vi "Digital_Bridge_3_kart.vi"() -> ()   [LabVIEW 2014] (continued)
                      frame True {
                        n3554 = local read "Frekanslar"() -> (w1876:dbl[])
                        n3555 = Array Size(array=w1876) -> (size(s)=w1875:i32)
                        n3556 = local read "frekans index"() -> (w1877:dbl)
                        n3557 = Decrement(x=w1875) -> (x-1=w1874:i32)
                        n3558 = Equal?(x=w1877, y=w1874) -> (x = y?=w1878:bool)
                        n3559 = case shown="False" w1878 {
                          tunnel: w1877 -> [w1879 w1891]
                          frame False {
                            n3560 = flat-sequence {
                              tunnel: w1879 -> [w1881]
                              frame #0 {
                                n3561 = local read "control hz array"() -> (w1883:dbl[][])
                                n3562 = call "change2d.vi"("reset(default false)"=FALSE, "index (col)"=w1881, "index (row)"=3, "read/write(T/F)"=FALSE, "2D Array"=w1883) -> ("2D Array Result"=w1882:dbl[][])  [unwired: 5 in, 1 out]
                                n3563 = local write "control hz array"(w1882) -> ()
                              }
                              frame #1 {
                                n3564 = local read "frekans index"() -> (w1890:dbl)
                                n3565 = local write "default input"(TRUE ("default values 2")) -> ()
                                n3566 = Increment(x=w1890) -> (x+1=w1889:dbl)
                                n3567 = local write "continue"(FALSE ("continue")) -> ()
                                n3568 = local write "error 2"(FALSE ("continue")) -> ()
                                n3569 = local write "frekans index"(w1889) -> ()
                              }
                            }
                          }
                          frame True {
                            n3570 = flat-sequence {
                              tunnel: w1891 -> [w1893]
                              frame #0 {
                                n3571 = local read "control hz array"() -> (w1895:dbl[][])
                                n3572 = call "change2d.vi"("reset(default false)"=FALSE, "index (col)"=w1893, "index (row)"=3, "read/write(T/F)"=FALSE, "2D Array"=w1895) -> ("2D Array Result"=w1894:dbl[][])  [unwired: 5 in, 1 out]
                                n3573 = local write "control hz array"(w1894) -> ()
                              }
                              frame #1 {
                                n3574 = local write "frekans index"(0.0 ("frekans index")) -> ()
                                n3575 = local write "default input"(TRUE ("default values 2")) -> ()
                                n3576 = local write "continue"(FALSE ("continue")) -> ()
                                n3577 = local write "error 2"(FALSE ("continue")) -> ()
                              }
                            }
                          }
                        }
                      }
                    }
                  }
                  frame True {
                    n3578 = local read "Frekanslar"() -> (w1904:dbl[])
                    n3579 = local read "frekans index"() -> (w1906:dbl)
                    n3580 = Array Size(array=w1904) -> (size(s)=w1903:i32)
                    n3581 = Decrement(x=w1903) -> (x-1=w1902:i32)
                    n3582 = Equal?(x=w1906, y=w1902) -> (x = y?=w1905:bool)
                    n3583 = case shown="True" w1905 {
                      frame False {
                        n3584 = flat-sequence {
                          frame #0 {
                            n3585 = local read "frekans index"() -> (w1908:dbl)
                            n3586 = Increment(x=w1908) -> (x+1=w1907:dbl)
                            n3587 = local write "frekans index"(w1907) -> ()
                          }
                          frame #1 {
                            n3588 = local write "default input"(TRUE ("default values 2")) -> ()
                            n3589 = local write "continue"(FALSE ("continue")) -> ()
                          }
                          frame #2 {
                            n3590 = local write "pass hz"(FALSE ("pass hz")) -> ()
                          }
                          frame #3 {
                          }
                        }
                      }
                      frame True {
                        n3591 = flat-sequence {
                          frame #0 {
                            n3592 = local write "frekans index"(0.0 ("frekans index")) -> ()
                          }
                          frame #1 {
                            n3593 = local write "default input"(TRUE ("default values 2")) -> ()
                            n3594 = local write "continue"(FALSE ("continue")) -> ()
                          }
                          frame #2 {
                            n3595 = local write "pass hz"(FALSE ("pass hz")) -> ()
                          }
                          frame #3 {
                          }
                        }
                      }
                    }
                  }
                }
              }
              frame #2 {
                w1916 = 0.0 ("amplitude 2/0")
                w1918 = 0.0 ("result output x [Wagner]")
                w1920 = FALSE ("Boolean 5")
                w1921 = FALSE
                w1922 = FALSE
                n3596 = case shown="True" "default input" {
                  frame False {
                  }
                  frame True {
                    n3597 = flat-sequence {
                      frame #0 {
                        w1936 = 0.0 ("iterasyon ana denge")
                        w1935 = 0.0 ("iterasyon ana denge")
                        w1934 = 0.0 ("iterasyon ana denge")
                        w1933 = 0.0 ("iterasyon ana denge")
                        w1932 = 0.0 ("iterasyon ana denge")
                        # "Frekans a göre iterasyon x algıla ona gore faz alınacak"
                        n3598 = global read "First_input_values.vi" "Active"() -> (w1923:bool)
                        n3599 = local read "frekans index"() -> (w1930:dbl)
                        n3600 = local read "control hz array"() -> (w1927:dbl[][])
                        n3601 = local write "output 1 y [10R]"(w1936) -> ()
                        n3602 = local write "input 1 y [10R]"(w1936) -> ()
                        n3603 = local write "output 2 y [10R]"(w1936) -> ()
                        n3604 = local write "input 2 y [10R]"(w1936) -> ()
                        n3605 = local write "input 2 x [10R]"(w1936) -> ()
                        n3606 = local write "output 2 x [10R]"(w1936) -> ()
                        n3607 = local write "input 1 x [10R]"(w1936) -> ()
                        n3608 = local write "output 1 x [10R]"(w1936) -> ()
                        n3609 = call "change2d.vi"("reset(default false)"=FALSE, "index (col)"=w1930, "index (row)"=3, "read/write(T/F)"=TRUE, "2D Array"=w1927) -> ("result count"=w1926:dbl)  [unwired: 5 in, 1 out]
                        n3610 = case shown="True" w1923 {
                          frame False {
                            n3611 = global read "First_input_values.vi" "X 1. input W"() -> (w1979:dbl)
                            n3612 = global read "First_input_values.vi" "X 2. input W"() -> (w1980:dbl)
                            n3613 = global read "First_input_values.vi" "X 1. input W"() -> (w1984:dbl)
                            n3614 = global read "First_input_values.vi" "X 2. input W"() -> (w1983:dbl)
                            n3615 = global read "First_input_values.vi" "Y 1. input W"() -> (w1981:dbl)
                            n3616 = global read "First_input_values.vi" "Y 2. input W"() -> (w1982:dbl)
                            n3617 = global read "First_input_values.vi" "Y 1. input W"() -> (w1986:dbl)
                            n3618 = global read "First_input_values.vi" "Y 2. input W"() -> (w1985:dbl)
                            n3619 = global read "First_input_values.vi" "X 1. input KV"() -> (w1971:dbl)
                            n3620 = global read "First_input_values.vi" "X 2. input KV"() -> (w1972:dbl)
                            n3621 = global read "First_input_values.vi" "X 1. input KV"() -> (w1976:dbl)
                            n3622 = global read "First_input_values.vi" "X 2. input KV"() -> (w1975:dbl)
                            n3623 = global read "First_input_values.vi" "Y 1. input KV"() -> (w1973:dbl)
                            n3624 = global read "First_input_values.vi" "Y 2. input KV"() -> (w1974:dbl)
                            n3625 = global read "First_input_values.vi" "Y 1. input KV"() -> (w1978:dbl)
                            n3626 = global read "First_input_values.vi" "Y 2. input KV"() -> (w1977:dbl)
                            n3627 = local write "Wagner Xk"(w1979) -> ()
                            n3628 = local write "Wagner  X(k-1)"(w1980) -> ()
                            n3629 = local write "X 1.input W"(w1984) -> ()
                            n3630 = local write "X 2.input W"(w1983) -> ()
                            n3631 = local write "Wagner Yk"(w1981) -> ()
                            n3632 = local write "Wagner Y(k-1)"(w1982) -> ()
                            n3633 = local write "Y 1.input W"(w1986) -> ()
                            n3634 = local write "Y 2.input W"(w1985) -> ()
                            n3635 = local write "Kelvin Xk"(w1971) -> ()
                            n3636 = local write "Kelvin X(k-1)"(w1972) -> ()
                            n3637 = local write "X 1.input KV"(w1976) -> ()
                            n3638 = local write "X 2.input KV"(w1975) -> ()
                            n3639 = local write "Kelvin Yk"(w1973) -> ()
                            n3640 = local write "Kelvin Y(k-1)"(w1974) -> ()
                            n3641 = local write "Y 1.input KV"(w1978) -> ()
                            n3642 = local write "Y 2.input KV"(w1977) -> ()
                            n3643 = global read "First_input_values.vi" "X 1. input AD"() -> (w1963:dbl)
                            n3644 = global read "First_input_values.vi" "X 2. input AD"() -> (w1964:dbl)
                            n3645 = global read "First_input_values.vi" "X 1. input AD"() -> (w1968:dbl)
                            n3646 = global read "First_input_values.vi" "X 2. input AD"() -> (w1967:dbl)
                            n3647 = global read "First_input_values.vi" "Y 1. input AD"() -> (w1965:dbl)
                            n3648 = global read "First_input_values.vi" "Y 2. input AD"() -> (w1966:dbl)
                            n3649 = global read "First_input_values.vi" "Y 1. input AD"() -> (w1970:dbl)
                            n3650 = global read "First_input_values.vi" "Y 2. input AD"() -> (w1969:dbl)
                            n3651 = global read "First_input_values.vi" "X 1. input 10R"() -> (w1955:dbl)
                            n3652 = global read "First_input_values.vi" "X 2. input 10R"() -> (w1956:dbl)
                            n3653 = global read "First_input_values.vi" "Y 1. input 10R"() -> (w1957:dbl)
                            n3654 = global read "First_input_values.vi" "Y 2. input 10R"() -> (w1958:dbl)
                            n3655 = global read "First_input_values.vi" "X 1. input 10R"() -> (w1960:dbl)
                            n3656 = global read "First_input_values.vi" "X 2. input 10R"() -> (w1959:dbl)
                            n3657 = global read "First_input_values.vi" "Y 1. input 10R"() -> (w1962:dbl)
                            n3658 = global read "First_input_values.vi" "Y 2. input 10R"() -> (w1961:dbl)
                            n3659 = local write "AD Xk"(w1963) -> ()
                            n3660 = local write "AD X(k-1)"(w1964) -> ()
                            n3661 = local write "X 1.input AD"(w1968) -> ()
                            n3662 = local write "X 2.input AD"(w1967) -> ()
                            n3663 = local write "AD Yk"(w1965) -> ()
                            n3664 = local write "AD Y(k-1)"(w1966) -> ()
                            n3665 = local write "Y 1.input AD"(w1970) -> ()
                            n3666 = local write "Y 2.input AD"(w1969) -> ()
                            n3667 = local write "10R Xk"(w1955) -> ()
                            n3668 = local write "10R X(k-1)"(w1956) -> ()
                            n3669 = local write "X 1.input 10R"(w1960) -> ()
                            n3670 = local write "X 2.input 10R"(w1959) -> ()
                            n3671 = local write "10R Yk"(w1957) -> ()
                            n3672 = local write "10R Y(k-1)"(w1958) -> ()
                            n3673 = local write "Y 1.input 10R"(w1962) -> ()
                            n3674 = local write "Y 2.input 10R"(w1961) -> ()
                            n3675 = global read "First_input_values.vi" "X 1. input 1R"() -> (w1947:dbl)
                            n3676 = global read "First_input_values.vi" "X 2. input 1R"() -> (w1948:dbl)
                            n3677 = global read "First_input_values.vi" "X 1. input 1R"() -> (w1952:dbl)
                            n3678 = global read "First_input_values.vi" "X 2. input 1R"() -> (w1951:dbl)
                            n3679 = global read "First_input_values.vi" "Y 1. input 1R"() -> (w1949:dbl)
                            n3680 = global read "First_input_values.vi" "Y 2. input 1R"() -> (w1950:dbl)
                            n3681 = global read "First_input_values.vi" "Y 1. input 1R"() -> (w1954:dbl)
                            n3682 = global read "First_input_values.vi" "Y 2. input 1R"() -> (w1953:dbl)
                            n3683 = global read "First_input_values.vi" "Y range 10R"() -> (w1945:dbl)
                            n3684 = global read "First_input_values.vi" "Y range AD"() -> (w1946:dbl)
                            n3685 = global read "First_input_values.vi" "X range 10R"() -> (w1940:dbl)
                            n3686 = global read "First_input_values.vi" "Y range KV"() -> (w1942:dbl)
                            n3687 = global read "First_input_values.vi" "Y range 1R"() -> (w1944:dbl)
                            n3688 = global read "First_input_values.vi" "X range AD"() -> (w1941:dbl)
                            n3689 = global read "First_input_values.vi" "Y range W"() -> (w1943:dbl)
                            n3690 = global read "First_input_values.vi" "X range KV"() -> (w1937:dbl)
                            n3691 = global read "First_input_values.vi" "X range 1R"() -> (w1939:dbl)
                            n3692 = global read "First_input_values.vi" "X range W"() -> (w1938:dbl)
                            n3693 = local write "1R Xk"(w1947) -> ()
                            n3694 = local write "1R X(k-1)"(w1948) -> ()
                            n3695 = local write "X 1.input 1R"(w1952) -> ()
                            n3696 = local write "X 2.input 1R"(w1951) -> ()
                            n3697 = local write "1R Yk"(w1949) -> ()
                            n3698 = local write "1R Y(k-1)"(w1950) -> ()
                            n3699 = local write "Y 1.input 1R"(w1954) -> ()
                            n3700 = local write "Y 2.input 1R"(w1953) -> ()
                            n3701 = local write "Y Range AD"(w1946) -> ()
                            n3702 = local write "Y Range 10R"(w1945) -> ()
                            n3703 = local write "Y Range 1R"(w1944) -> ()
                            n3704 = local write "Y Range W"(w1943) -> ()
                            n3705 = local write "Y Range KV"(w1942) -> ()
                            n3706 = local write "X Range AD"(w1941) -> ()
                            n3707 = local write "X Range 10R"(w1940) -> ()
                            n3708 = local write "X Range 1R"(w1939) -> ()
                            n3709 = local write "X Range W"(w1938) -> ()
                            n3710 = local write "X Range KV"(w1937) -> ()
                          }
                          frame True {
                            n3711 = for {
                              N: 6 -> [_]
                              i -> [w1989]
                              n3712 = for {
                                N: 5 -> [_]
                                tunnel: w1989 -> [w1993]
                                i -> [w1992]
                                n3713 = local read "frekans index"() -> (w1990:dbl)
                                n3714 = global read "First_input_values.vi" "Multi Values"() -> (w1994:dbl[][][])
                                n3715 = Index Array(array=w1994, index (dim 0)=w1990, index (dim 1)=w1993, index (dim 2)=w1992) -> (element=w1991:dbl)
                                n3716 = case shown="0, Default" w1993 {
                                tunnel: w1992 -> [w1996 w2003 w2010 w2017 w2024 w2031]
                                tunnel: w1991 -> [w1995 w2002 w2009 w2016 w2023 w2030]
                                frame 0, Default {
                                n3717 = case shown="2" w1996 {
                                tunnel: w1995 -> [w1997 w1998 w1999 w2000 w2001]
                                frame 0, Default {
                                n3718 = local write "X 1.input AD"(w1997) -> ()
                                n3719 = local write "AD Xk"(w1997) -> ()
                                }
                                frame 1 {
                                n3720 = local write "X 1.input 10R"(w1998) -> ()
                                n3721 = local write "10R Xk"(w1998) -> ()
                                }
                                frame 2 {
                                n3722 = local write "1R Xk"(w1999) -> ()
                                n3723 = local write "X 1.input 1R"(w1999) -> ()
                                }
                                frame 3 {
                                n3724 = local write "Wagner Xk"(w2000) -> ()
                                n3725 = local write "X 1.input W"(w2000) -> ()
                                }
                                frame 4 {
                                n3726 = local write "Kelvin Xk"(w2001) -> ()
                                n3727 = local write "X 1.input KV"(w2001) -> ()
                                }
                                }
                                }
                                frame 1 {
                                n3728 = case shown="1" w2003 {
                                tunnel: w2002 -> [w2004 w2005 w2006 w2007 w2008]
                                frame 0, Default {
                                n3729 = local write "AD X(k-1)"(w2004) -> ()
                                n3730 = local write "X 2.input AD"(w2004) -> ()
                                }
                                frame 1 {
                                n3731 = local write "10R X(k-1)"(w2005) -> ()
                                n3732 = local write "X 2.input 10R"(w2005) -> ()
                                }
                                frame 2 {
                                n3733 = local write "1R X(k-1)"(w2006) -> ()
                                n3734 = local write "X 2.input 1R"(w2006) -> ()
                                }
                                frame 3 {
                                n3735 = local write "Wagner  X(k-1)"(w2007) -> ()
                                n3736 = local write "X 2.input W"(w2007) -> ()
                                }
                                frame 4 {
                                n3737 = local write "Kelvin X(k-1)"(w2008) -> ()
                                n3738 = local write "X 2.input KV"(w2008) -> ()
                                }
                                }
                                }
                                frame 2 {
                                n3739 = case shown="4" w2010 {
                                tunnel: w2009 -> [w2011 w2012 w2013 w2014 w2015]
                                frame 0, Default {
                                n3740 = local write "X Range AD"(w2011) -> ()
                                }
                                frame 1 {
                                n3741 = local write "X Range 10R"(w2012) -> ()
                                }
                                frame 2 {
                                n3742 = local write "X Range 1R"(w2013) -> ()
                                }
                                frame 3 {
                                n3743 = local write "X Range W"(w2014) -> ()
                                }
                                frame 4 {
                                n3744 = local write "X Range KV"(w2015) -> ()
                                }
                                }
                                }
                                frame 3 {
                                n3745 = case shown="4" w2017 {
                                tunnel: w2016 -> [w2018 w2019 w2020 w2021 w2022]
                                frame 0, Default {
                                n3746 = local write "AD Yk"(w2018) -> ()
                                n3747 = local write "Y 1.input AD"(w2018) -> ()
                                }
                                frame 1 {
                                n3748 = local write "10R Yk"(w2019) -> ()
                                n3749 = local write "Y 1.input 10R"(w2019) -> ()
                                }
                                frame 2 {
                                n3750 = local write "1R Yk"(w2020) -> ()
                                n3751 = local write "Y 1.input 1R"(w2020) -> ()
                                }
                                frame 3 {
                                n3752 = local write "Wagner Yk"(w2021) -> ()
                                n3753 = local write "Y 1.input W"(w2021) -> ()
                                }
                                frame 4 {
                                n3754 = local write "Kelvin Yk"(w2022) -> ()
                                n3755 = local write "Y 1.input KV"(w2022) -> ()
                                }
                                }
                                }
                                frame 4 {
                                n3756 = case shown="2" w2024 {
                                tunnel: w2023 -> [w2025 w2026 w2027 w2028 w2029]
                                frame 0, Default {
                                n3757 = local write "AD Y(k-1)"(w2025) -> ()
                                n3758 = local write "Y 2.input AD"(w2025) -> ()
                                }
                                frame 1 {
                                n3759 = local write "10R Y(k-1)"(w2026) -> ()
                                n3760 = local write "Y 2.input 10R"(w2026) -> ()
                                }
                                frame 2 {
                                n3761 = local write "1R Y(k-1)"(w2027) -> ()
                                n3762 = local write "Y 2.input 1R"(w2027) -> ()
                                }
                                frame 3 {
                                n3763 = local write "Wagner Y(k-1)"(w2028) -> ()
                                n3764 = local write "Y 2.input W"(w2028) -> ()
                                }
                                frame 4 {
                                n3765 = local write "Kelvin Y(k-1)"(w2029) -> ()
                                n3766 = local write "Y 2.input KV"(w2029) -> ()
                                }
                                }
                                }
                                frame 5 {
                                n3767 = case shown="0, Default" w2031 {
                                tunnel: w2030 -> [w2032 w2033 w2034 w2035 w2036]
                                frame 0, Default {
                                n3768 = local write "Y Range AD"(w2032) -> ()
                                }
                                frame 1 {
                                n3769 = local write "Y Range 10R"(w2033) -> ()
                                }
                                frame 2 {
                                n3770 = local write "Y Range 1R"(w2034) -> ()
                                }
                                frame 3 {
                                n3771 = local write "Y Range W"(w2035) -> ()
                                }
                                frame 4 {
                                n3772 = local write "Y Range W"(w2036) -> ()
                                }
                                }
                                }
                                }
                              }
                            }
                          }
                        }
                        n3773 = Greater?(x=w1926, y=0.0) -> (0:w1924:bool)
                        n3774 = case shown="False" w1924 {
                          frame False {
                            n3775 = local read "Direnc 1 - Direnc 2"() -> (w2046:u32)
                            n3776 = local read "Wagner F/P Array"() -> (w2042:dbl[][])
                            n3777 = local read "Kelvin F/P Array"() -> (w2043:dbl[][])
                            n3778 = local read "10R F/P Array"() -> (w2040:dbl[][])
                            n3779 = local read "frekans index"() -> (w2045:dbl)
                            n3780 = local read "AD F/P Array"() -> (w2039:dbl[][])
                            n3781 = local read "1R F/P Array"() -> (w2041:dbl[][])
                            n3782 = local read "Frekanslar"() -> (w2044:dbl[])
                            n3783 = control-ref of="Default Values Listbox"() -> (w2038:refnum<vi>)
                            n3784 = Increment(x=w2046) -> (x+1=w2047:u32)
                            n3785 = call "check 5 phase.vi"("LstBox Refnum"=w2038, "AD F/P Array"=w2039, "10R F/P Array"=w2040, "1R F/P Array"=w2041, "Wagner F/P Array"=w2042, "Kelvin F/P Array"=w2043, "Direnc 1 - Direnc 2"=w2047, "Frekanslar"=w2044, "frekans index"=w2045) -> ("logical AND"=w2037:bool)  [unwired: 10 in]
                            n3786 = case shown="False" w2037 {
                              frame False {
                                w2048 = 1.0 ("iterasyon ana denge")
                                w2049 = 1.0 ("iterasyon ana denge")
                                n3787 = local write "İterasyon Y 5"(w2049) -> ()
                                n3788 = local write "İterasyon X 5"(w2049) -> ()
                                n3789 = local write "İterasyon Y 4"(w2049) -> ()
                                n3790 = local write "İterasyon X 4"(w2049) -> ()
                                n3791 = local write "İterasyon Y 3"(w2049) -> ()
                                n3792 = local write "İterasyon X 3"(w2049) -> ()
                                n3793 = local write "İterasyon Y 2"(w2049) -> ()
                                n3794 = local write "İterasyon X 2"(w2049) -> ()
                                n3795 = local write "İterasyon Y"(w2049) -> ()
                                n3796 = local write "İterasyon X"(w2049) -> ()
                                n3797 = local write "iterasyon 10R"(w2048) -> ()
                                n3798 = local write "iterasyon 1R"(w2048) -> ()
                                n3799 = local write "iterasyon WAGNER"(w2048) -> ()
                                n3800 = local write "iterasyon KELVIN"(w2048) -> ()
                                n3801 = local write "iterasyon AD"(w2048) -> ()
                              }
                              frame True {
                                w2050 = 0.0 ("iterasyon ana denge")
                                w2051 = 0.0 ("iterasyon ana denge")
                                n3802 = local write "İterasyon Y 5"(w2051) -> ()
                                n3803 = local write "İterasyon X 5"(w2051) -> ()
                                n3804 = local write "İterasyon Y 4"(w2051) -> ()
                                n3805 = local write "İterasyon X 4"(w2051) -> ()
                                n3806 = local write "İterasyon Y 3"(w2051) -> ()
                                n3807 = local write "İterasyon X 3"(w2051) -> ()
                                n3808 = local write "İterasyon Y 2"(w2051) -> ()
                                n3809 = local write "İterasyon X 2"(w2051) -> ()
                                n3810 = local write "İterasyon Y"(w2051) -> ()
                                n3811 = local write "İterasyon X"(w2051) -> ()
                                n3812 = local write "iterasyon 10R"(w2050) -> ()
                                n3813 = local write "iterasyon 1R"(w2050) -> ()
                                n3814 = local write "iterasyon WAGNER"(w2050) -> ()
                                n3815 = local write "iterasyon KELVIN"(w2050) -> ()
                                n3816 = local write "iterasyon AD"(w2050) -> ()
                              }
                            }
                          }
                          frame True {
                            w2052 = 0.0 ("iterasyon ana denge")
                            w2053 = 0.0 ("iterasyon ana denge")
                            n3817 = local write "İterasyon Y 5"(w2053) -> ()
                            n3818 = local write "İterasyon X 5"(w2053) -> ()
                            n3819 = local write "İterasyon Y 4"(w2053) -> ()
                            n3820 = local write "İterasyon X 4"(w2053) -> ()
                            n3821 = local write "İterasyon Y 3"(w2053) -> ()
                            n3822 = local write "İterasyon X 3"(w2053) -> ()
                            n3823 = local write "İterasyon Y 2"(w2053) -> ()
                            n3824 = local write "İterasyon X 2"(w2053) -> ()
                            n3825 = local write "İterasyon Y"(w2053) -> ()
                            n3826 = local write "İterasyon X"(w2053) -> ()
                            n3827 = local write "iterasyon 10R"(w2052) -> ()
                            n3828 = local write "iterasyon 1R"(w2052) -> ()
                            n3829 = local write "iterasyon WAGNER"(w2052) -> ()
                            n3830 = local write "iterasyon KELVIN"(w2052) -> ()
                            n3831 = local write "iterasyon AD"(w2052) -> ()
                          }
                        }
                        n3832 = local write "output 1 y [ana denge]"(w1935) -> ()
                        n3833 = local write "output 2 y [ana denge]"(w1935) -> ()
                        n3834 = local write "input 2 y [ana denge]"(w1935) -> ()
                        n3835 = local write "input 1 y [ana denge]"(w1935) -> ()
                        n3836 = local write "input 2 x [ana denge]"(w1935) -> ()
                        n3837 = local write "input 1 x [ana denge]"(w1935) -> ()
                        n3838 = local write "output 1 x [ana denge]"(w1935) -> ()
                        n3839 = local write "output 2 x [ana denge]"(w1935) -> ()
                        n3840 = local write "output 2 y [wagner]"(w1933) -> ()
                        n3841 = local write "output 1 y [wagner]"(w1933) -> ()
                        n3842 = local write "input 2 y [wagner]"(w1933) -> ()
                        n3843 = local write "input 1 y [wagner]"(w1933) -> ()
                        n3844 = local write "output 2 x [wagner]"(w1933) -> ()
                        n3845 = local write "output 1 x [wagner]"(w1933) -> ()
                        n3846 = local write "input 2 x [wagner]"(w1933) -> ()
                        n3847 = local write "input 1 x [wagner]"(w1933) -> ()
                        n3848 = local write "output 2 y [kelvin]"(w1934) -> ()
                        n3849 = local write "output 1 y [kelvin]"(w1934) -> ()
                        n3850 = local write "input 2 y [kelvin]"(w1934) -> ()
                        n3851 = local write "input 1 y [kelvin]"(w1934) -> ()
                        n3852 = local write "output 1 x [kelvin]"(w1934) -> ()
                        n3853 = local write "output 2 x [kelvin]"(w1934) -> ()
                        n3854 = local write "input 2 x [kelvin]"(w1934) -> ()
                        n3855 = local write "input 1 x [kelvin]"(w1934) -> ()
                        n3856 = local write "output 2 y [1R]"(w1932) -> ()
                        n3857 = local write "output 1 y [1R]"(w1932) -> ()
                        n3858 = local write "input 2 y [1R]"(w1932) -> ()
                        n3859 = local write "input 1 y [1R]"(w1932) -> ()
                        n3860 = local write "input 2 x [1R]"(w1932) -> ()
                        n3861 = local write "input 1 x [1R]"(w1932) -> ()
                        n3862 = local write "output 1 x [1R]"(w1932) -> ()
                        n3863 = local write "output 2 x [1R]"(w1932) -> ()
                      }
                      frame #1 {
                        n3864 = local write "default input"(FALSE) -> ()
                      }
                    }
                  }
                }
                n3865 = local write "KONTROL Y"(w1922) -> ()
                n3866 = local write "KONTROL X"(w1922) -> ()
                n3867 = local write "KONTROL Y 5"(w1922) -> ()
                n3868 = local write "KONTROL X 5"(w1922) -> ()
                n3869 = local write "KONTROL Y 3"(w1922) -> ()
                n3870 = local write "KONTROL X 2"(w1922) -> ()
                n3871 = local write "KONTROL Y 2"(w1922) -> ()
                n3872 = local write "KONTROL X 3"(w1922) -> ()
                n3873 = local write "KONTROL Y 4"(w1922) -> ()
                n3874 = local write "KONTROL X 4"(w1922) -> ()
                n3875 = local write "X"(w1922) -> ()
                n3876 = local write "RANGE KONTROL X 5"(w1922) -> ()
                n3877 = local write "Y"(w1922) -> ()
                n3878 = local write "RANGE KONTROL X 2"(w1922) -> ()
                n3879 = local write "X 2"(w1922) -> ()
                n3880 = local write "RANGE KONTROL X 3"(w1922) -> ()
                n3881 = local write "Y 2"(w1922) -> ()
                n3882 = local write "RANGE KONTROL Y 5"(w1922) -> ()
                n3883 = local write "X 3"(w1922) -> ()
                n3884 = local write "RANGE KONTROL Y"(w1922) -> ()
                n3885 = local write "Y 3"(w1922) -> ()
                n3886 = local write "Iterasyon Successful"(0.0 ("Iterasyon Successful")) -> ()
                n3887 = local write "PASS 10R"(w1921) -> ()
                n3888 = local write "PASS 1R"(w1921) -> ()
                n3889 = local write "PASS ANA D"(w1921) -> ()
                n3890 = local write "PASS KELVIN"(w1921) -> ()
                n3891 = local write "PASS WAGNER"(w1921) -> ()
                n3892 = local write "X1"(w1922) -> ()
                n3893 = local write "IF ELSE X 5"(w1922) -> ()
                n3894 = local write "Y1"(w1922) -> ()
                n3895 = local write "IF ELSE Y 4"(w1922) -> ()
                n3896 = local write "X1 2"(w1922) -> ()
                n3897 = local write "IF ELSE Y 5"(w1922) -> ()
                n3898 = local write "Y1 2"(w1922) -> ()
                n3899 = local write "IF ELSE Y"(w1922) -> ()
                n3900 = local write "X1 3"(w1922) -> ()
                n3901 = local write "IF ELSE X"(w1922) -> ()
                n3902 = local write "Y1 3"(w1922) -> ()
                n3903 = local write "result output y [Kelvin]"(w1918) -> ()
                n3904 = local write "result output x [Kelvin]"(w1918) -> ()
                n3905 = local write "result output y [AD]"(w1918) -> ()
                n3906 = local write "result output x [AD]"(w1918) -> ()
                n3907 = local write "result output y [10R]"(w1918) -> ()
                n3908 = local write "result output x [10R]"(w1918) -> ()
                n3909 = local write "result output y [1R]"(w1918) -> ()
                n3910 = local write "result output x [1R]"(w1918) -> ()
                n3911 = local write "result output y [Wagner]"(w1918) -> ()
                n3912 = local write "result output x [Wagner]"(w1918) -> ()
                n3913 = local write "RANGE KONTROL X"(w1922) -> ()
                n3914 = local write "Y 4"(w1922) -> ()
                n3915 = local write "RANGE KONTROL Y 2"(w1922) -> ()
                n3916 = local write "Y"(w1922) -> ()
                n3917 = local write "RANGE KONTROL Y 3"(w1922) -> ()
                n3918 = local write "X 5"(w1922) -> ()
                n3919 = local write "RANGE KONTROL X 4"(w1922) -> ()
                n3920 = local write "Y 5"(w1922) -> ()
                n3921 = local write "RANGE KONTROL Y 4"(w1922) -> ()
                n3922 = global write "DB_Global_4_kart-Test.vi" "amplitude 2/0"(w1916) -> ()
                n3923 = global write "DB_Global_4_kart-Test.vi" "phase 2/ 0"(w1916) -> ()
                n3924 = global write "DB_Global_4_kart-Test.vi" "amplitude 3/0"(w1916) -> ()
                n3925 = global write "DB_Global_4_kart-Test.vi" "phase 3/0"(w1916) -> ()
                n3926 = global write "DB_Global_4_kart-Test.vi" "amplitude 1/1"(w1916) -> ()
                n3927 = global write "DB_Global_4_kart-Test.vi" "phase 1/1"(w1916) -> ()
                n3928 = global write "DB_Global_4_kart-Test.vi" "amplitude 2/1"(w1916) -> ()
                n3929 = global write "DB_Global_4_kart-Test.vi" "phase 2/1"(w1916) -> ()
                n3930 = global write "DB_Global_4_kart-Test.vi" "amplitude 3/1"(w1916) -> ()
                n3931 = global write "DB_Global_4_kart-Test.vi" "phase 3/1"(w1916) -> ()
                n3932 = local write "Boolean"(w1920) -> ()
                n3933 = local write "Boolean 4"(w1920) -> ()
                n3934 = local write "Boolean 2"(w1920) -> ()
                n3935 = local write "Boolean 3"(w1920) -> ()
                n3936 = local write "Boolean 5"(w1920) -> ()
                n3937 = local write "IF ELSE Y 2"(w1922) -> ()
                n3938 = local write "X1 4"(w1922) -> ()
                n3939 = local write "IF ELSE X 2"(w1922) -> ()
                n3940 = local write "Y1 4"(w1922) -> ()
                n3941 = local write "IF ELSE Y 3"(w1922) -> ()
                n3942 = local write "X1 5"(w1922) -> ()
                n3943 = local write "IF ELSE X 3"(w1922) -> ()
                n3944 = local write "Y1 5"(w1922) -> ()
                n3945 = local write "IF ELSE X 4"(w1922) -> ()
              }
              frame #3 {
                n3946 = Wait (ms)(milliseconds to wait=u32 250) -> ()  [unwired: 1 out]
              }
              frame #4 {
                n3947 = local read "count meas"() -> (w2073:u16)
                n3948 = Greater?(x=w2073, y=u16 8) -> (0:w2071:bool)
                n3949 = case shown="True" "continue" {
                  frame False {
                  }
                  frame True {
                    n3950 = flat-sequence {
                      frame #0 {
                        n3951 = local read "default values"() -> (w4138:T3)
                        n3952 = local read "frekans index"() -> (w4139:dbl)
                        n3953 = Index Array(array=w4138, index=w4139) -> (element=w4137:T12)
                        n3954 = Unbundle By Name(w4137) -> ("Ana Denge Xk"=w4136:dbl, "10R Xk"=w4135:dbl, "1R Xk"=w4134:dbl, "Wagner Xk"=w4133:dbl, "Kelvin Xk"=w4132:dbl, "Ana Denge Xk-1"=w4131:dbl, "10R Xk-1"=w4130:dbl, "1R Xk-1"=w4129:dbl, "Wagner Xk-1"=w4128:dbl, "Kelvin Xk-1"=w4127:dbl, "Ana Denge Yk"=w4126:dbl, "10R Yk"=w4125:dbl, "1R Yk"=w4124:dbl, "Wagner Yk"=w4123:dbl, "Kelvin Yk"=w4122:dbl, "Ana Denge Yk-1"=w4121:dbl, "10R Yk-1"=w4120:dbl, "1R Yk-1"=w4119:dbl, "Wagner Yk-1"=w4118:dbl, "Kelvin Yk-1"=w4117:dbl)
                        n3955 = local write "AD Xk"(w4136) -> ()
                        n3956 = local write "10R Xk"(w4135) -> ()
                        n3957 = local write "1R Xk"(w4134) -> ()
                        n3958 = local write "Wagner Xk"(w4133) -> ()
                        n3959 = local write "Kelvin Xk"(w4132) -> ()
                        n3960 = local write "AD X(k-1)"(w4131) -> ()
                        n3961 = local write "10R X(k-1)"(w4130) -> ()
                        n3962 = local write "1R X(k-1)"(w4129) -> ()
                        n3963 = local write "Wagner  X(k-1)"(w4128) -> ()
                        n3964 = local write "Kelvin X(k-1)"(w4127) -> ()
                        n3965 = local write "AD Yk"(w4126) -> ()
                        n3966 = local write "10R Yk"(w4125) -> ()
                        n3967 = local write "1R Yk"(w4124) -> ()
                        n3968 = local write "Wagner Yk"(w4123) -> ()
                        n3969 = local write "Kelvin Yk"(w4122) -> ()
                        n3970 = local write "AD Y(k-1)"(w4121) -> ()
                        n3971 = local write "10R Y(k-1)"(w4120) -> ()
                        n3972 = local write "1R Y(k-1)"(w4119) -> ()
                        n3973 = local write "Wagner Y(k-1)"(w4118) -> ()
                        n3974 = local write "Kelvin Y(k-1)"(w4117) -> ()
                      }
                      frame #1 {
                        n3975 = Wait (ms)(milliseconds to wait=u32 500) -> ()  [unwired: 1 out]
                      }
                      frame #2 {
                        n3976 = local read "Wagner Xk"() -> (w4148:dbl)
                        n3977 = local read "Wagner Yk"() -> (w4147:dbl)
                        n3978 = local read "10R Xk"() -> (w4146:dbl)
                        n3979 = local read "10R Yk"() -> (w4145:dbl)
                        n3980 = local read "AD Xk"() -> (w4150:dbl)
                        n3981 = local read "AD Yk"() -> (w4149:dbl)
                        n3982 = local read "Kelvin Xk"() -> (w4141:dbl)
                        n3983 = local read "Kelvin Yk"() -> (w4142:dbl)
                        n3984 = local read "1R Xk"() -> (w4144:dbl)
                        n3985 = local read "1R Yk"() -> (w4143:dbl)
                        n3986 = global write "DB_Global_4_kart-Test.vi" "amplitude 2/0"(w4150) -> ()
                        n3987 = global write "DB_Global_4_kart-Test.vi" "phase 2/ 0"(w4149) -> ()
                        n3988 = global write "DB_Global_4_kart-Test.vi" "amplitude 3/0"(w4146) -> ()
                        n3989 = global write "DB_Global_4_kart-Test.vi" "phase 3/0"(w4145) -> ()
                        n3990 = global write "DB_Global_4_kart-Test.vi" "amplitude 1/1"(w4148) -> ()
                        n3991 = global write "DB_Global_4_kart-Test.vi" "phase 1/1"(w4147) -> ()
                        n3992 = global write "DB_Global_4_kart-Test.vi" "amplitude 2/1"(w4141) -> ()
                        n3993 = global write "DB_Global_4_kart-Test.vi" "phase 2/1"(w4142) -> ()
                        n3994 = global write "DB_Global_4_kart-Test.vi" "amplitude 3/1"(w4144) -> ()
                        n3995 = global write "DB_Global_4_kart-Test.vi" "phase 3/1"(w4143) -> ()
                      }
                      frame #3 {
                        n3996 = local write "dummy fix default"(FALSE ("continue")) -> ()
                        n3997 = local write "continue"(FALSE ("continue")) -> ()
                      }
                    }
                  }
                }
                n3998 = case shown="True" w2071 {
                  frame False {
                  }
                  frame True {
                    n3999 = local read "count meas"() -> (w2174:u16)
                    n4000 = Equal?(x=w2174, y=u16 10) -> (x = y?=w2173:bool)
                    n4001 = case shown="False" w2173 {
                      frame False {
                        n4002 = local read "frekans index"() -> (w2179:dbl)
                        n4003 = flat-sequence {
                          tunnel: w2176 -> [w2188]
                          tunnel: [w2188] -> w2181
                          tunnel: w2181 -> [w2506]
                          tunnel: [w2506] -> w2180
                          tunnel: w2180 -> [w2824]
                          frame #0 {
                            n4004 = local read "Denge Seçimi"() -> (w2189:u8)
                            n4005 = case shown="5" w2189 {
                              tunnel: w2188 -> [w2190 w2254 w2318 w2382 w2442]
                              frame 1 {
                                n4006 = for {
                                N: 10 -> [_]
                                tunnel: w2190 -> [w2192]
                                i -> [w2195]
                                n4007 = local read "Denge Kosulu x2_y2"() -> (w2194:dbl[][])
                                n4008 = case shown="5" w2195 {
                                tunnel: w2195 -> [w2196 w2203 w2214 w2219 w2224 w2229 w2234 w2239 w2244 w2248]
                                tunnel: w2194 -> [w2197 w2205 w2213 w2218 w2223 w2228 w2232 w2237 w2245 w2249]
                                tunnel: [w2198 w2206 w2211 w2217 w2222 w2227 w2231 w2236 w2246 w2250] -> w2193
                                tunnel: w2192 -> [w2199 w2204 w2212 w2216 w2221 w2226 w2233 w2238 w2243 w2247]
                                frame 0, Default {
                                n4009 = Index Array(array=w2197, index (row)=w2196, index (col)=w2199) -> (element=w2202:dbl)
                                n4010 = Multiply(x=w2202, y=2.0) -> (x*y=w2200:dbl)
                                n4011 = Replace Array Subset(array=w2197, new element=w2200, index (row)=w2196, index (col)=w2199) -> (w2198:dbl[][])
                                }
                                frame 1 {
                                n4012 = Index Array(array=w2205, index (row)=w2203, index (col)=w2204) -> (element=w2209:dbl)
                                n4013 = Multiply(x=w2209, y=2.0) -> (x*y=w2207:dbl)
                                n4014 = Replace Array Subset(array=w2205, new element=w2207, index (row)=w2203, index (col)=w2204) -> (w2206:dbl[][])
                                }
                                frame 2 {
                                n4015 = Index Array(array=w2213, index (row)=w2214, index (col)=w2212) -> (element=w2210:dbl)
                                n4016 = Replace Array Subset(array=w2213, new element=w2210, index (row)=w2214, index (col)=w2212) -> (w2211:dbl[][])
                                }
                                frame 3 {
                                n4017 = Index Array(array=w2218, index (row)=w2219, index (col)=w2216) -> (element=w2215:dbl)
                                n4018 = Replace Array Subset(array=w2218, new element=w2215, index (row)=w2219, index (col)=w2216) -> (w2217:dbl[][])
                                }
                                frame 4 {
                                n4019 = Index Array(array=w2223, index (row)=w2224, index (col)=w2221) -> (element=w2220:dbl)
                                n4020 = Replace Array Subset(array=w2223, new element=w2220, index (row)=w2224, index (col)=w2221) -> (w2222:dbl[][])
                                }
                                frame 5 {
                                n4021 = Index Array(array=w2228, index (row)=w2229, index (col)=w2226) -> (element=w2225:dbl)
                                n4022 = Replace Array Subset(array=w2228, new element=w2225, index (row)=w2229, index (col)=w2226) -> (w2227:dbl[][])
                                }
                                frame 6 {
                                n4023 = Index Array(array=w2232, index (row)=w2234, index (col)=w2233) -> (element=w2230:dbl)
                                n4024 = Replace Array Subset(array=w2232, new element=w2230, index (row)=w2234, index (col)=w2233) -> (w2231:dbl[][])
                                }
                                frame 7 {
                                n4025 = Index Array(array=w2237, index (row)=w2239, index (col)=w2238) -> (element=w2235:dbl)
                                n4026 = Replace Array Subset(array=w2237, new element=w2235, index (row)=w2239, index (col)=w2238) -> (w2236:dbl[][])
                                }
                                frame 8 {
                                n4027 = Index Array(array=w2245, index (row)=w2244, index (col)=w2243) -> (element=w2242:dbl)
                                n4028 = Multiply(x=w2242, y=2.0) -> (x*y=w2240:dbl)
                                n4029 = Replace Array Subset(array=w2245, new element=w2240, index (row)=w2244, index (col)=w2243) -> (w2246:dbl[][])
                                }
                                frame 9 {
                                n4030 = Index Array(array=w2249, index (row)=w2248, index (col)=w2247) -> (element=w2253:dbl)
                                n4031 = Multiply(x=w2253, y=2.0) -> (x*y=w2251:dbl)
                                n4032 = Replace Array Subset(array=w2249, new element=w2251, index (row)=w2248, index (col)=w2247) -> (w2250:dbl[][])
                                }
                                }
                                n4033 = local write "Denge Kosulu x2_y2"(w2193) -> ()
                                }
                              }
                              frame 2 {
                                n4034 = for {
                                N: 10 -> [_]
                                tunnel: w2254 -> [w2256]
                                i -> [w2259]
                                n4035 = local read "Denge Kosulu x2_y2"() -> (w2258:dbl[][])
                                n4036 = case shown="7" w2259 {
                                tunnel: w2259 -> [w2261 w2266 w2273 w2280 w2287 w2294 w2302 w2307 w2310 w2315]
                                tunnel: w2258 -> [w2262 w2268 w2272 w2279 w2286 w2293 w2300 w2305 w2311 w2316]
                                tunnel: [w2263 w2269 w2270 w2278 w2285 w2292 w2299 w2304 w2312 w2317] -> w2257
                                tunnel: w2256 -> [w2264 w2267 w2271 w2277 w2284 w2291 w2301 w2306 w2309 w2314]
                                frame 0, Default {
                                n4037 = Index Array(array=w2262, index (row)=w2261, index (col)=w2264) -> (element=w2260:dbl)
                                n4038 = Replace Array Subset(array=w2262, new element=w2260, index (row)=w2261, index (col)=w2264) -> (w2263:dbl[][])
                                }
                                frame 1 {
                                n4039 = Index Array(array=w2268, index (row)=w2266, index (col)=w2267) -> (element=w2265:dbl)
                                n4040 = Replace Array Subset(array=w2268, new element=w2265, index (row)=w2266, index (col)=w2267) -> (w2269:dbl[][])
                                }
                                frame 2 {
                                n4041 = Index Array(array=w2272, index (row)=w2273, index (col)=w2271) -> (element=w2276:dbl)
                                n4042 = Multiply(x=w2276, y=2.0) -> (x*y=w2274:dbl)
                                n4043 = Replace Array Subset(array=w2272, new element=w2274, index (row)=w2273, index (col)=w2271) -> (w2270:dbl[][])
                                }
                                frame 3 {
                                n4044 = Index Array(array=w2279, index (row)=w2280, index (col)=w2277) -> (element=w2283:dbl)
                                n4045 = Multiply(x=w2283, y=2.0) -> (x*y=w2281:dbl)
                                n4046 = Replace Array Subset(array=w2279, new element=w2281, index (row)=w2280, index (col)=w2277) -> (w2278:dbl[][])
                                }
                                frame 4 {
                                n4047 = Index Array(array=w2286, index (row)=w2287, index (col)=w2284) -> (element=w2290:dbl)
                                n4048 = Multiply(x=w2290, y=2.0) -> (x*y=w2288:dbl)
                                n4049 = Replace Array Subset(array=w2286, new element=w2288, index (row)=w2287, index (col)=w2284) -> (w2285:dbl[][])
                                }
                                frame 5 {
                                n4050 = Index Array(array=w2293, index (row)=w2294, index (col)=w2291) -> (element=w2297:dbl)
                                n4051 = Multiply(x=w2297, y=2.0) -> (x*y=w2295:dbl)
                                n4052 = Replace Array Subset(array=w2293, new element=w2295, index (row)=w2294, index (col)=w2291) -> (w2292:dbl[][])
                                }
                                frame 6 {
                                n4053 = Index Array(array=w2300, index (row)=w2302, index (col)=w2301) -> (element=w2298:dbl)
                                n4054 = Replace Array Subset(array=w2300, new element=w2298, index (row)=w2302, index (col)=w2301) -> (w2299:dbl[][])
                                }
                                frame 7 {
                                n4055 = Index Array(array=w2305, index (row)=w2307, index (col)=w2306) -> (element=w2303:dbl)
                                n4056 = Replace Array Subset(array=w2305, new element=w2303, index (row)=w2307, index (col)=w2306) -> (w2304:dbl[][])
                                }
                                frame 8 {
                                n4057 = Index Array(array=w2311, index (row)=w2310, index (col)=w2309) -> (element=w2308:dbl)
                                n4058 = Replace Array Subset(array=w2311, new element=w2308, index (row)=w2310, index (col)=w2309) -> (w2312:dbl[][])
                                }
                                frame 9 {
